vi "Main UI.vi"() -> ()   [LabVIEW 2013]
uses:
  <vilib>/Utility/miscctls.llb/LVRowAndColumnTypeDef.ctl
  <vilib>/Utility/miscctls.llb/LVRowAndColumnUnsignedTypeDef.ctl
  Sub vi/Global constant.vi
  <vilib>/regexp/Match Regular Expression.xnode
panel:
  out "Operator":string="A1644"
  out "W/O Qty":string="20000"
  out "Work Order":string="1644"
  out "Date Code (YYWW)":string="4416" caption="D/C (YYWW)"
  out "Lot Number (6 digits)":string="123456" caption="L/N (6 digits)"
  out "Part Number_Die Ver_Field":string="206CAH" caption="P/N_Die Ver_Field"
  out "FPY":cluster{"fail":u32, "pass":u32, "FPY":dbl}={"fail"=12345, "pass"=1234567, "FPY"=0.0} caption="FPY (Pass/Fail/Rate %)"
  out "Test Time":string
  in  "Cancel Button":bool
  out "SN":string
  out "Model":string
  out "Result":string
  in  "OK Button":bool
  in  "Multicolumn Listbox":i32(listbox)
  out "Horizontal Graduated Bar":u8(slide) max=28 scale=-1.0..7.0
  in  "Boolean 2":bool
  out "reslut":bool
  out "Boolean":bool
  out "?":string[](array[string])
  out "ItemTag":string
  # "Melexis Auto-Programming Machine\nFor MLX91206"
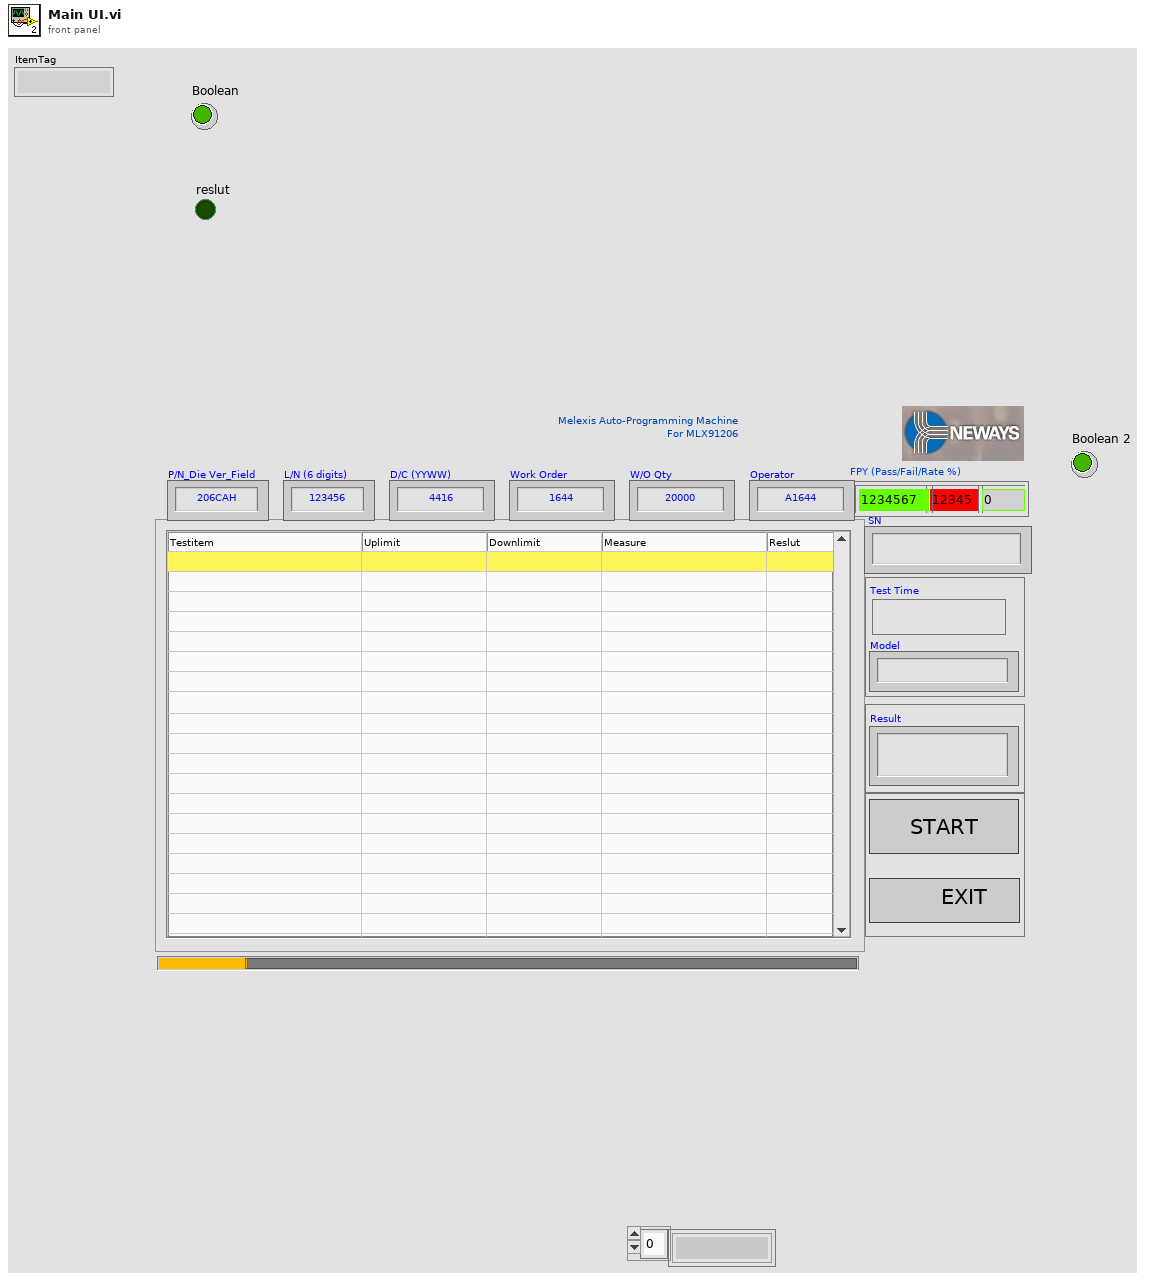
[diagram p1: front panel]
types:
  T1 = enum8{"Enabled", "Disabled", "Disabled and Grayed Out"}
  T2 = enum16{"open", "replace", "create", "open or create", "replace or create", "replace or create with confirmation"}
  T3 = typedef "LVRowAndColumnUnsignedTypeDef.ctl" = cluster{"Row":u32, "Column":u32}
  T4 = typedef "LVRowAndColumnTypeDef.ctl" = cluster{"Row":i32, "Column":i32}
  T5 = cluster{"step name 1":string, "updata 2":string, "limitdata 3":string, "load vi name 4":string, "parameter 5":string}
  T6 = cluster{"concatenated string":string, "Result":bool}
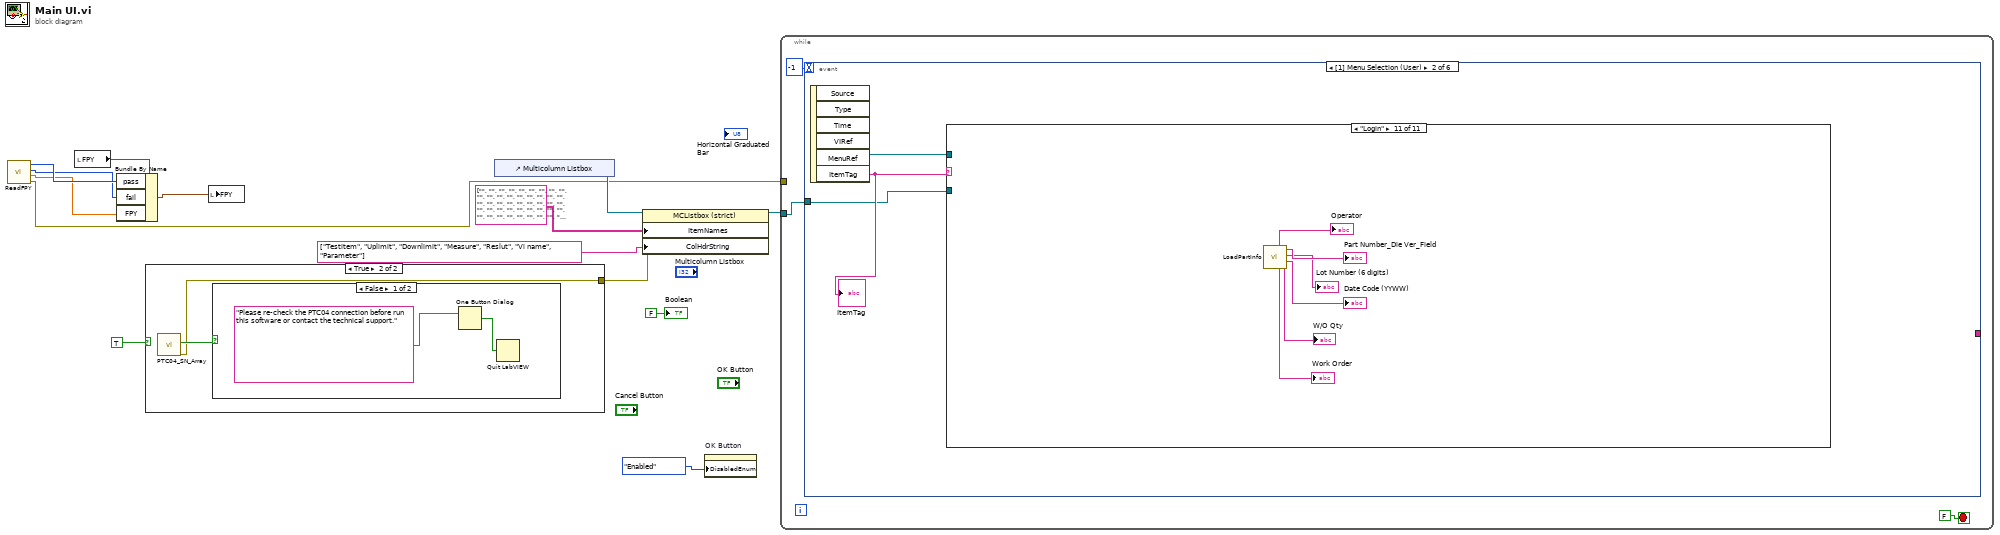
[diagram p0: block diagram]
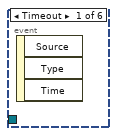
[diagram p4: hidden frame]
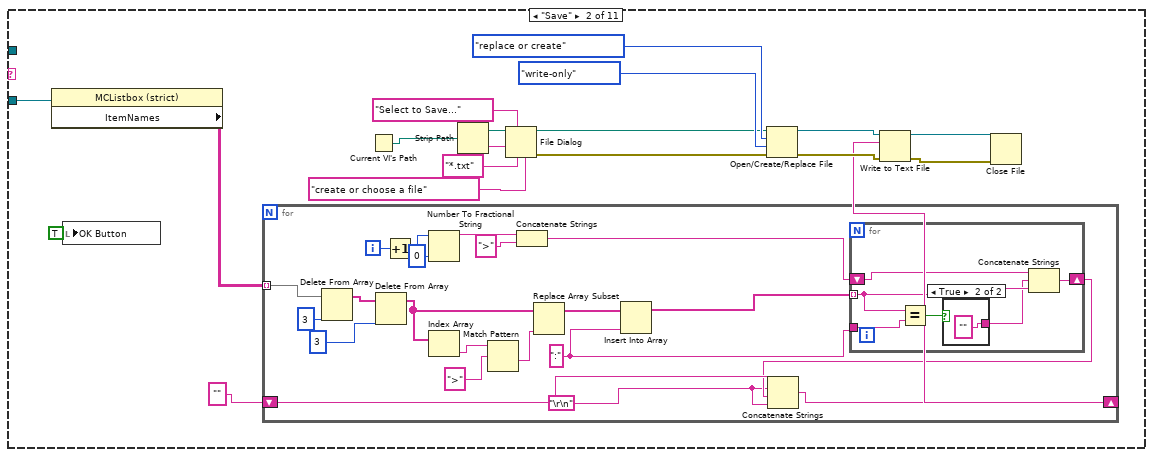
[diagram p6: hidden frame]
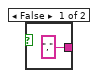
[diagram p7: hidden frame]
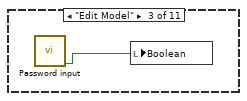
[diagram p8: hidden frame]
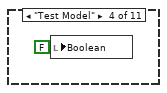
[diagram p9: hidden frame]
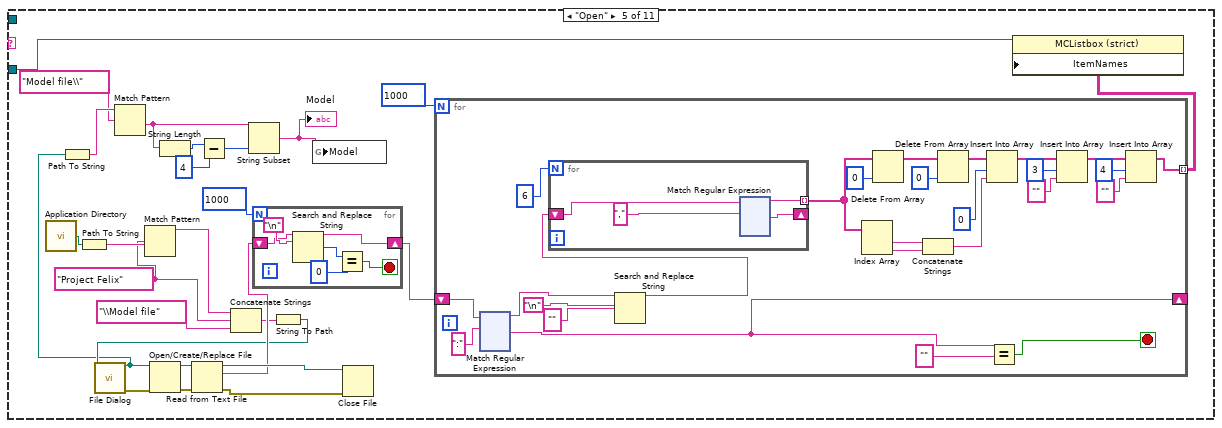
[diagram p10: hidden frame]
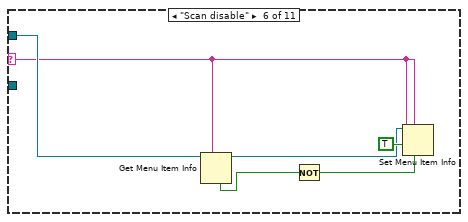
[diagram p11: hidden frame]
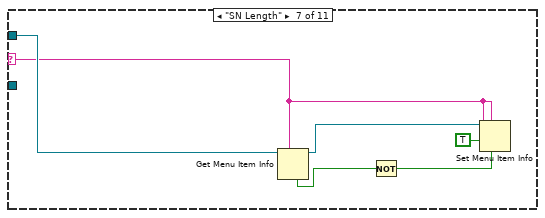
[diagram p12: hidden frame]
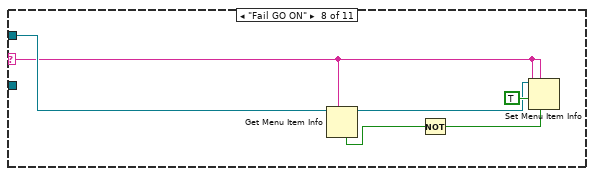
[diagram p13: hidden frame]
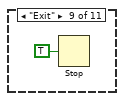
[diagram p14: hidden frame]
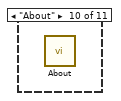
[diagram p15: hidden frame]
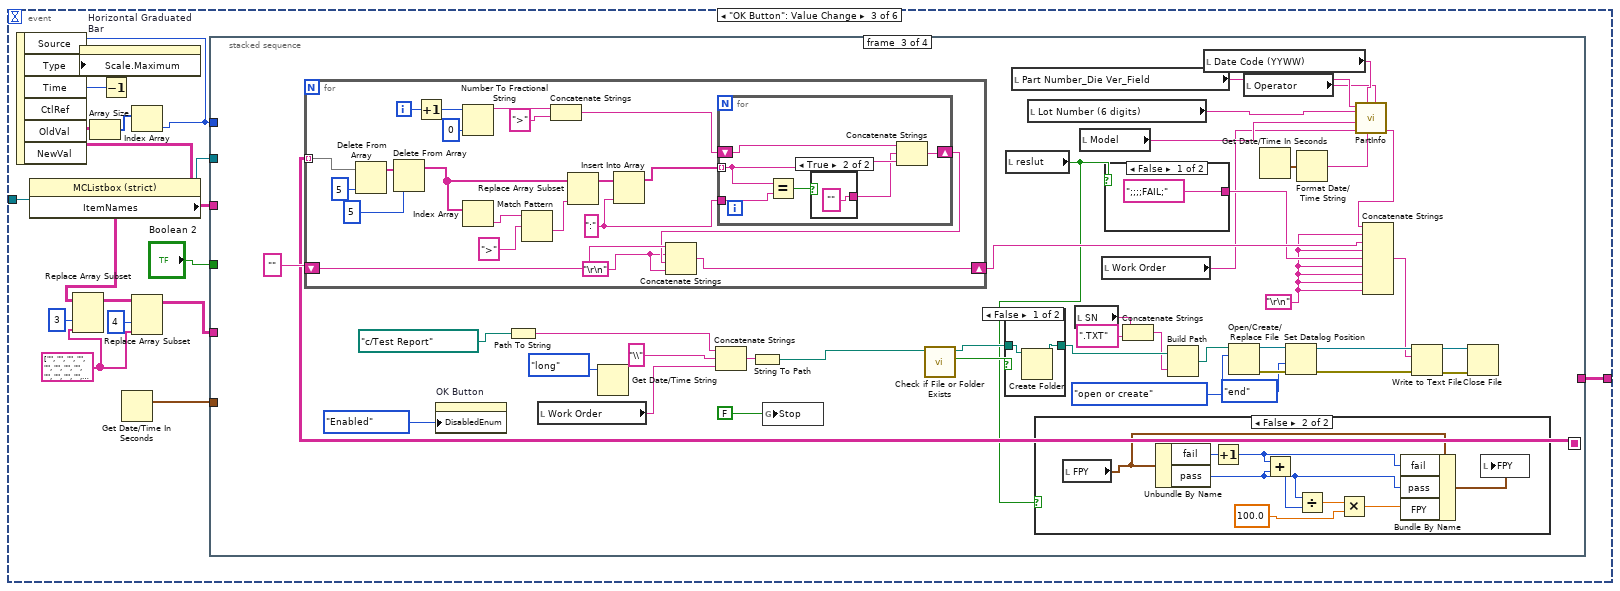
[diagram p16: hidden frame]
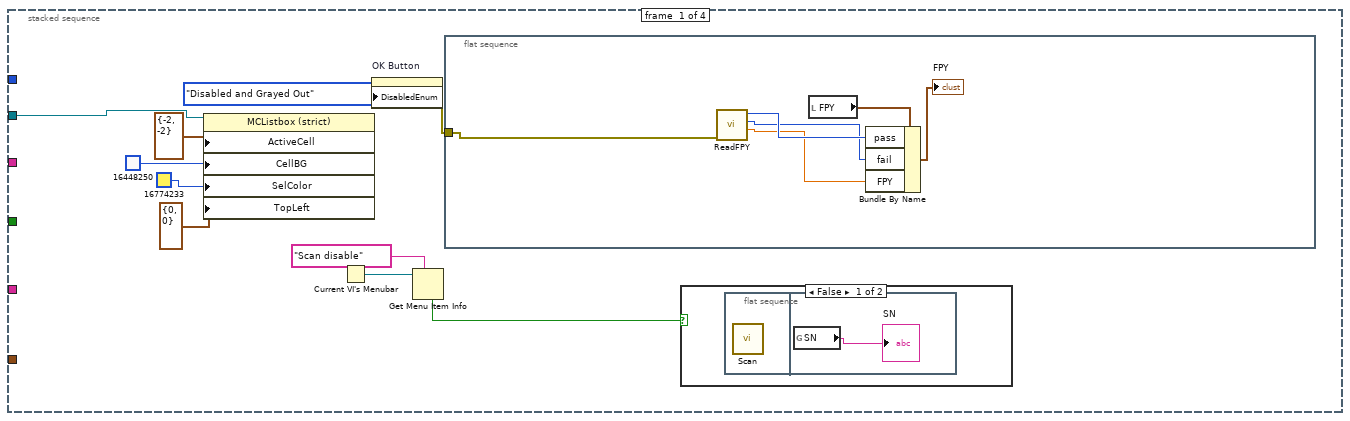
[diagram p17: hidden frame]
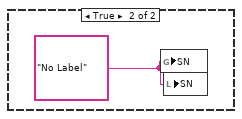
[diagram p18: hidden frame]
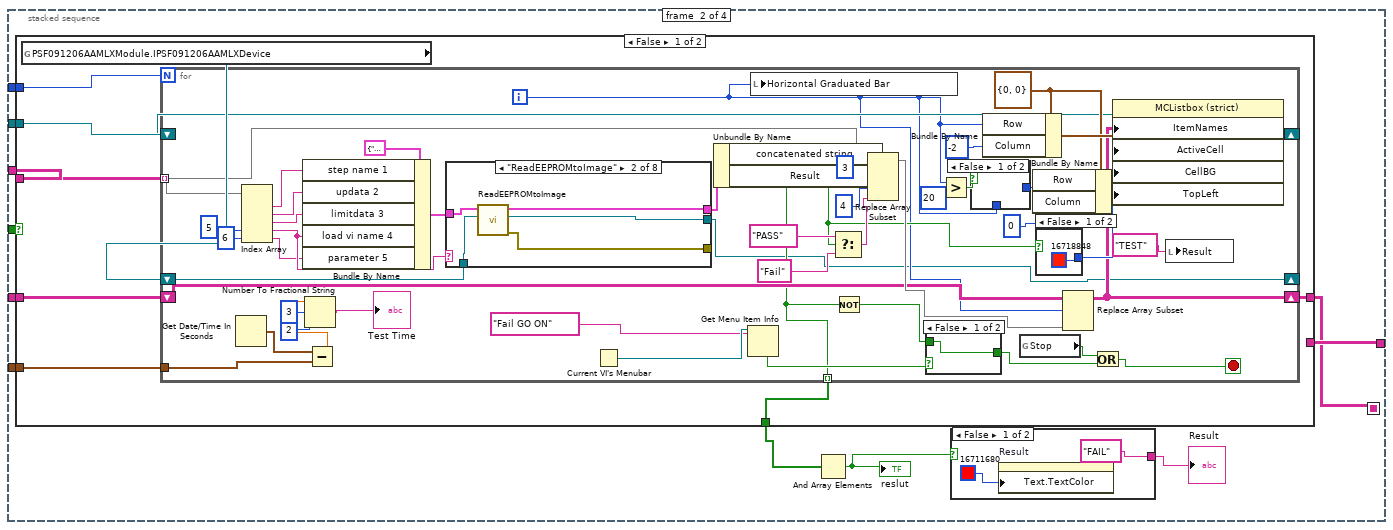
[diagram p19: hidden frame]
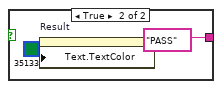
[diagram p20: hidden frame]
diagram:
  n1 = call "ReadFPY.vi"() -> ("error out"=w1:errorcluster, "FPY%"=w3:dbl, "fail"=w4:i32, "pass"=w5:i32)  [unwired: 7 in, 1 out]
  n2 = local read "FPY"() -> (w6:cluster{"fail":u32, "pass":u32, "FPY":dbl})
  n3 = Bundle By Name(cluster=w6, "pass"=w5, "fail"=w4, "FPY"=w3) -> (w2:cluster{"fail":u32, "pass":u32, "FPY":dbl})
  n4 = case shown="True" TRUE {
    tunnel: [_ w15] -> w7
    frame False {
    }
    frame True {
      n5 = call "PTC04_SN_Array.vi"() -> ("error out"=w15:errorcluster, "Register?"=w16:bool)  [unwired: 9 in, 1 out]
      n6 = case shown="False" w16 {
        frame False {
          n7 = One Button Dialog(message="Please re-check the PTC04 connection before run this software or contact the technical support.") -> (true=w17:bool)  [unwired: 1 in]
          n8 = Quit LabVIEW(quit? (T)=w17) -> ()
        }
        frame True {
        }
      }
    }
  }
  n9 = local write "FPY"(w2) -> ()
  n10 = control-ref of="Multicolumn Listbox"() -> (w14:refnum<vi>)
  n11 = property class="MCListbox (strict)"(reference=w14, error in=w7, "ItemNames"=string[][] [["", "", "", "", "", "", "", ""], ["", "", "", "", "", "", "", ""], ["", "", "", "", "", "", "", ""], ["", "", "", "", "", "", "", ""], ["", "", "", "", "", "", "", ""], ["", "", "", "", "", "", "", ""], ["", "", "", "", "", "", "", ""], ["", "", "", "", "", "", "", ""], ["", "", "", "", "", "", "", ""], ["", "", "", "", "", "", "", ""], ["", "", "", "", "", "", "", ""], ["", "", "", "", "", "", "", ""], ["", "", "", "", "", "", "", ""], ["", "", "", "", "", "", "", ""], ["", "", "", "", "", "", "", ""], ["", "", "", "", "", "", "", ""], ["", "", "", "", "", "", "", ""], ["", "", "", "", "", "", "", ""], ["", "", "", "", "", "", "", ""], ["", "", "", "", "", "", "", ""], ["", "", "", "", "", "", "", ""], ["", "", "", "", "", "", "", " "], ["", "", "", "", "", "", "", ""], ["", "", "", "", "", "", "", ""], ["", "", "", "", "", "", "", ""], ["", "", "", "", "", "", "", ""], ["", "", "", "", "", "", "", ""], ["", "", "", "", "", "", "", ""], ["", "", "", "", "", "", "", ""], ["", "", "", "", "", "", "", ""], ["", "", "", "", "", "", "", ""], ["", "", "", "", "", "", "", ""], ["", "", "", "", "", "", "", ""], ["", "", "", "", "", "", "", ""], ["", "", "", "", "", "", "", ""], ["", "", "", "", "", "", "", ""], ["", "", "", "", "", "", "", ""], ["", "", "", "", "", "", "", ""], ["", "", "", "", "", "", "", ""], ["", "", "", "", "", "", "", ""], ["", "", "", "", "", "", "", ""], ["", "", "", "", "", "", "", ""]] ("Item Names"), "ColHdrString"=string[] ["Testitem", "Uplimit", "Downlimit", "Measure", "Reslut", "Vi name", "Parameter"] ("Row Header Strings[]")) -> (reference out=w11:refnum<vi>)  [unwired: 1 out]
  n12 = property on="OK Button" class="Bool (strict)"("DisabledEnum"=T1."Enabled" ("Disabled")) -> ()  [unwired: 2 in, 2 out]
  n13 = while {
    tunnel: w11 -> [w21]
    tunnel: w1 -> [_]
    stop <- FALSE stop-if-true
    n14 = event shown="[1] Menu Selection (User)" {
      selector: _ -> [_ _ _ _ _ _]
      dyn-events: _ -> [_ _ _ _ _ _]
      timeout: -1 -> [_ _ _ _ _ _]
      tunnel: w21 -> [_ w23 w403 _ w712 w735]
      tunnel: [_ _ w390 _ _ _] -> _
      event Timeout {
        n15 = event-data() -> ()  [unwired: 1 in, 3 out]
      }
      event Menu Selection (User) {
        n16 = event-data() -> ("MenuRef"=w22:refnum<k9>, "ItemTag"=w24:string)  [unwired: 1 in, 4 out]
        "ItemTag" <- w24
        n17 = case shown="\"Login\"" w24 {
          selector: w24 -> [_ _ _ _ _ w365 w371 w380 _ _ _]
          tunnel: w23 -> [_ w43 _ _ w96 _ _ _ _ _ _]
          tunnel: w22 -> [_ _ _ _ _ w366 w372 w381 _ _ _]
          frame "False", Default {
          }
          frame "Save" {
            n18 = property class="MCListbox (strict)"(reference=w43) -> ("ItemNames"=w32:string[][])  [unwired: 1 in, 2 out]
            n19 = local write "OK Button"(TRUE ("OK Button")) -> ()
            n20 = for {
              tunnel: w32 -> [w54] mode=indexing
              shift-right: [w58] -> w29
              shift-left: "" -> [w57]
              i -> [w64]
              w44 = ":" ("new element/subarray")
              w55 = "\r\n"
              n21 = Delete From Array(array=w54, index=3) -> (array with subset deleted=w51:string[])  [unwired: 1 in, 1 out]
              n22 = Delete From Array(array=w51, index=3) -> (array with subset deleted=w49:string[])  [unwired: 1 in, 1 out]
              n23 = Increment(x=w64) -> (x+1=w63:i32)
              n24 = Number To Fractional String(number=w63, precision (6)=i16 0) -> (F-format string=w62:string)  [unwired: 2 in]
              n25 = Index Array(array=w49) -> (element=w50:string)  [unwired: 1 in]
              n26 = Match Pattern(string=w50, regular expression=">") -> (after substring=w48:string)  [unwired: 1 in, 3 out]
              n27 = Concatenate Strings(w62, ">") -> (w60:string)
              n28 = Replace Array Subset(array=w49, new element=w48) -> (w46:string[])  [unwired: 1 in]
              n29 = Insert Into Array(array=w46, new element=w44) -> (w45:string[])  [unwired: 1 in]
              n30 = for {
                shift-right: [w69] -> w56
                shift-left: w60 -> [w70]
                tunnel: w45 -> [w67] mode=indexing
                tunnel: w44 -> [w68]
                n31 = Equal?(x=w67, y=w68) -> (x = y?=w66:bool)
                n32 = case shown="True" w66 {
                  tunnel: ["," ("string") ""] -> w65
                  frame False {
                  }
                  frame True {
                  }
                }
                n33 = Concatenate Strings(w70, w65, w67) -> (w69:string)
              }
              n34 = Concatenate Strings(w57, w55, w56, w55) -> (w58:string)
            }
            n35 = Current VI's Path() -> (path=w26:path)
            n36 = Strip Path(path=w26) -> (stripped path=w34:path, name=w35:string)
            n37 = File Dialog(4:"create or choose a file" ("pattern label"), 6:"*.txt" ("pattern (all files)"), 7:"Select to Save..." ("prompt"), 9:w35, 11:w34) -> (0:w37:errorcluster, 3:w36:path)  [unwired: 1 in, 3 out]
            n38 = Open/Create/Replace File(file path (use dialog)=w36, error in=w37, operation (0:open)=T2."replace or create", access (0:read/write)=enum16{"read/write", "read-only", "write-only"}."write-only") -> (refnum out=w30:refnum<file>, error out=w31:errorcluster)  [unwired: 3 out]
            n39 = Write to Text File(file (use dialog)=w30, text=w29, error in=w31) -> (refnum out=w27:refnum<file>, error out=w28:errorcluster)  [unwired: 1 in, 1 out]
            n40 = Close File(refnum=w27, error in=w28) -> ()  [unwired: 2 out]
          }
          frame "Edit Model" {
            n41 = call "Password input.vi"() -> ("Boolean"=w73:bool)  [unwired: 10 in, 1 out]
            n42 = local write "Boolean"(w73) -> ()
          }
          frame "Test Model" {
            n43 = local write "Boolean"(FALSE ("Boolean")) -> ()
          }
          frame "Open" {
            w79 = "Project Felix" ("search string")
            n44 = call <vilib>:"Application Directory.vi"() -> ("Application Directory"=w82:path)
            n45 = Path To String(path=w82) -> (string=w81:string)
            n46 = Match Pattern(string=w81, regular expression=w79) -> (before substring=w80:string)  [unwired: 1 in, 3 out]
            n47 = Concatenate Strings(w80, w79, "\\Model file" ("string")) -> (w77:string)
            n48 = String To Path(string=w77) -> (path=w76:path)
            n49 = call "File Dialog"("start path"=w76) -> ("selected path"=w75:path, "error out"=w98:errorcluster)  [unwired: 11 in, 2 out]
            n50 = Path To String(path=w75) -> (string=w92:string)
            n51 = Match Pattern(string=w92, regular expression="Model file\\") -> (after substring=w87:string)  [unwired: 1 in, 3 out]
            n52 = Open/Create/Replace File(file path (use dialog)=w75, error in=w98) -> (refnum out=w99:refnum<file>, error out=w100:errorcluster)  [unwired: 4 in, 1 out]
            n53 = String Length(string=w87) -> (length=w90:i32)
            n54 = Read from Text File(file (use dialog)=w99, error in=w100) -> (refnum out=w93:refnum<file>, text=w85:string, error out=w94:errorcluster)  [unwired: 2 in, 1 out]
            n55 = Subtract(x=w90, y=4) -> (x-y=w88:i32)
            n56 = String Subset(string=w87, length (rest)=w88) -> (substring=w83:string)  [unwired: 1 in]
            "Model" <- w83
            n57 = for {
              N: 1000 -> [_]
              shift-right: [w104] -> w84
              shift-left: w85 -> [w105]
              stop <- w101 stop-if-true
              n58 = Search and Replace String(input string=w105, search string="\n") -> (result string=w104:string, number of replacements=w103:i32)  [unwired: 6 in, 2 out]
              n59 = Equal?(x=w103, y=0) -> (x = y?=w101:bool)
            }
            n60 = global write "Global constant.vi" "Model"(w83) -> ()
            n61 = Close File(refnum=w93, error in=w94) -> ()  [unwired: 2 out]
            n62 = for {
              N: 1000 -> [_]
              shift-right: [w113] -> _
              shift-left: w84 -> [w132]
              tunnel: [w114] -> w95 mode=indexing
              stop <- w111 stop-if-true
              n63 = xnode ("Match Regular Expression")("input string"=w132, "regular expression"=":") -> ("before match"=w110:string, "after match"=w113:string)  [unwired: 4 in, 3 out]
              n64 = Search and Replace String(input string=w110, search string="\n" ("Line Feed Constant"), replace string="" ("replace string (\"\")")) -> (result string=w107:string)  [unwired: 5 in, 3 out]
              n65 = for {
                N: 6 -> [_]
                shift-right: [w134] -> _
                shift-left: w107 -> [w135]
                tunnel: [w133] -> w127 mode=indexing
                n66 = xnode "Match Regular Expression"("input string"=w135, "regular expression"=",") -> ("before match"=w133:string, "after match"=w134:string)  [unwired: 4 in, 3 out]
              }
              n67 = Index Array(array=w127) -> (element #1=w128:string, element #2=w129:string)  [unwired: 2 in]
              n68 = Delete From Array(array=w127, index=0) -> (array with subset deleted=w126:string[])  [unwired: 1 in, 1 out]
              n69 = Concatenate Strings(w128, w129) -> (w122:string)
              n70 = Delete From Array(array=w126, index=0) -> (array with subset deleted=w123:string[])  [unwired: 1 in, 1 out]
              n71 = Insert Into Array(array=w123, index=0, new element=w122) -> (w120:string[])
              n72 = Equal?(x=w113, y="") -> (x = y?=w111:bool)
              n73 = Insert Into Array(array=w120, index=3, new element="" ("new element/subarray")) -> (w117:string[])
              n74 = Insert Into Array(array=w117, index=4, new element="" ("new element/subarray")) -> (w114:string[])
            }
            n75 = property class="MCListbox (strict)"(reference=w96, "ItemNames"=w95) -> ()  [unwired: 1 in, 2 out]
          }
          frame "Scan disable" {
            n76 = Get Menu Item Info(7:w365, 11:w366) -> (3:w367:refnum<k9>, 4:w369:bool)  [unwired: 1 in, 5 out]
            n77 = Not(x=w369) -> (.not. x?=w368:bool)
            n78 = Set Menu Item Info(6:w368, 7:w365, 9:TRUE ("enabled"), 10:w365, 11:w367) -> ()  [unwired: 2 in, 2 out]
          }
          frame "SN Length" {
            n79 = Get Menu Item Info(7:w371, 11:w372) -> (3:w373:refnum<k9>, 4:w375:bool)  [unwired: 1 in, 5 out]
            n80 = Not(x=w375) -> (.not. x?=w374:bool)
            n81 = Set Menu Item Info(6:w374, 7:w371, 9:TRUE ("enabled"), 10:w371, 11:w373) -> ()  [unwired: 2 in, 2 out]
          }
          frame "Fail GO ON" {
            n82 = Get Menu Item Info(7:w380, 11:w381) -> (3:w377:refnum<k9>, 4:w379:bool)  [unwired: 1 in, 5 out]
            n83 = Not(x=w379) -> (.not. x?=w378:bool)
            n84 = Set Menu Item Info(6:w378, 7:w380, 9:TRUE ("enabled"), 10:w380, 11:w377) -> ()  [unwired: 2 in, 2 out]
          }
          frame "Exit" {
            n85 = Stop(stop? (T)=TRUE) -> ()
          }
          frame "About" {
            n86 = call "About.vi"() -> ()  [unwired: 12 in]
          }
          frame "Login" {
            n87 = call "LoadPartInfo.vi"() -> ("W/O Qty"=→"W/O Qty":string, "Date Code (YYWW) 2"=→"Date Code (YYWW)":string, "Lot Number (6 digits) 2"=→"Lot Number (6 digits)":string, "Part Number_Die Ver_Field 2"=→"Part Number_Die Ver_Field":string, "Work Order 2"=→"Work Order":string, "Operator 2"=→"Operator":string)  [unwired: 6 in]
          }
        }
      }
      event "OK Button": Value Change {
        w400 = string[] ["", "", "", "", "", "", "", "", "", "", "", "", "", "", "", "", "", "", "", "", "", "", "", "", "", "", "", "", "", "", "", "", "", "", "", "", "", "", "", "", "", "", "", "", "", "", "", "", "", "", "", "", "", "", "", "", "", "", "", "", "", "", "", "", "", "", "", "", "", "", "", "", "", "", "", "", "", "", "", "", "", "", "", "", "", "", "", "", "", "", "", "", "", "", "", "", "", "", "", "", ""] ("new element/subarray")
        n88 = event-data() -> ()  [unwired: 1 in, 6 out]
        n89 = property class="MCListbox (strict)"(reference=w403) -> (reference out=w402:refnum<vi>, "ItemNames"=w395:string[][])  [unwired: 1 in, 1 out]
        n90 = Replace Array Subset(array=w395, new element=w400, index (col)=3 ("disabled index (col)")) -> (w399:string[][])  [unwired: 1 in]
        n91 = Array Size(array=w395) -> (size(s)=w396:i32[])
        n92 = Get Date/Time In Seconds() -> (seconds since 1Jan1904=w391:timestamp)
        n93 = Index Array(array=w396) -> (element=w392:i32)  [unwired: 1 in]
        n94 = Decrement(x=w392) -> (x-1=w393:i32)
        n95 = property on="Horizontal Graduated Bar" class="Slide (strict)"("Scale.Maximum"=w393) -> ()  [unwired: 2 in, 2 out]
        n96 = Replace Array Subset(array=w399, new element=w400, index (col)=4 ("disabled index (col)")) -> (w397:string[][])  [unwired: 1 in]
        n97 = stacked-sequence {
          seq-local: [_ w425 _ _] -> [_ _ w626 _]
          tunnel: w402 -> [w409 w429 _ _]
          tunnel: w392 -> [_ w432 _ _]
          tunnel: w397 -> [_ w431 _ _]
          tunnel: w395 -> [_ w430 _ _]
          tunnel: "Boolean 2" -> [_ w428 _ _]
          tunnel: w391 -> [_ w427 _ _]
          tunnel: [_ w426 _ _] -> w390
          frame #0 {
            n98 = property class="MCListbox (strict)"(reference=w409, "ActiveCell"=T4 {"Row"=-2, "Column"=-2} ("Active Cell:Active Cell"), "CellBG"=u32 16448250, "SelColor"=u32 16774233, "TopLeft"=T3 {"Row"=0, "Column"=0} ("Top Left Visible Cell")) -> ()  [unwired: 1 in, 2 out]
            n99 = Current VI's Menubar() -> (w412:refnum<k9>)
            n100 = property on="OK Button" class="Bool (strict)"("DisabledEnum"=T1."Disabled and Grayed Out" ("Disabled")) -> (error out=w404:errorcluster)  [unwired: 2 in, 1 out]
            n101 = Get Menu Item Info(7:"Scan disable" ("item tag"), 11:w412) -> (4:w410:bool)  [unwired: 1 in, 6 out]
            n102 = flat-sequence {
              tunnel: w404 -> [w417]
              frame #0 {
                n103 = call "ReadFPY.vi"("error in (no error)"=w417) -> ("FPY%"=w414:dbl, "fail"=w415:i32, "pass"=w416:i32)  [unwired: 6 in, 2 out]
                n104 = local read "FPY"() -> (w419:cluster{"fail":u32, "pass":u32, "FPY":dbl})
                n105 = Bundle By Name(cluster=w419, "pass"=w416, "fail"=w415, "FPY"=w414) -> (→"FPY":cluster{"fail":u32, "pass":u32, "FPY":dbl})
              }
            }
            n106 = case shown="False" w410 {
              frame False {
                n107 = flat-sequence {
                  frame #0 {
                    n108 = call "Scan.vi"() -> ()  [unwired: 12 in]
                  }
                  frame #1 {
                    n109 = global read "Global constant.vi" "SN"() -> (→"SN":string)
                  }
                }
              }
              frame True {
                w421 = "No Label"
                n110 = global write "Global constant.vi" "SN"(w421) -> ()
                n111 = local write "SN"(w421) -> ()
              }
            }
          }
          frame #1 {
            n112 = case shown="False" w428 {
              tunnel: w432 -> [w441 w545]
              tunnel: w431 -> [w444 w544]
              tunnel: w430 -> [w443 w543]
              tunnel: w429 -> [w442 w542]
              tunnel: [w440 w541] -> w422
              tunnel: w427 -> [w439 w540]
              tunnel: [_ w539] -> w426
              tunnel: [w438 _] -> w425
              frame False {
                n113 = global read "Global constant.vi" "PSF091206AAMLXModule.IPSF091206AAMLXDevice"() -> (w437:refnum<k7>)
                n114 = for {
                  N: w441 -> [_]
                  tunnel: w443 -> [w468] mode=indexing
                  shift-right: [w466] -> w438
                  shift-left: w444 -> [w467]
                  shift-right: [w465] -> _
                  shift-left: w442 -> [w469]
                  tunnel: [w462] -> w440 mode=indexing
                  tunnel: w439 -> [w459]
                  shift-right: [w446] -> _
                  shift-left: w437 -> [w445]
                  i -> [w461]
                  stop <- w449 stop-if-true
                  w476 = T4 {"Row"=0, "Column"=0} ("Active Cell:Active Cell")
                  n115 = Get Date/Time In Seconds() -> (seconds since 1Jan1904=w458:timestamp)
                  n116 = Index Array(array=w468, index #4=5 ("index"), index #5=6 ("index")) -> (element #1=w492:string, element #2=w491:string, element #3=w490:string, element #4=w453:string, element #5=w452:string)  [unwired: 3 in]
                  n117 = Bundle By Name(cluster=T5 {"step name 1"="", "updata 2"="", "limitdata 3"="", "load vi name 4"="", "parameter 5"=""} ("IN"), "step name 1"=w492, "updata 2"=w491, "limitdata 3"=w490, "load vi name 4"=w453, "parameter 5"=w452) -> (w489:T5)
                  n118 = Subtract(x=w458, y=w459) -> (x-y=w457:dbl)
                  n119 = Number To Fractional String(number=w457, width (-)=i16 3, precision (6)=i16 2) -> (F-format string=→"Test Time":string)  [unwired: 1 in]
                  n120 = case shown="\"ReadEEPROMtoImage\"" w453 {
                    tunnel: w489 -> [w504 w509 w513 w516 w521 w528 w533 w538]
                    tunnel: [w503 w508 w512 w518 w523 w526 w531 w536] -> _
                    tunnel: [w502 w507 w511 w517 w522 w527 w532 w537] -> w470
                    tunnel: [w501 w506 w510 w514 w520 w525 w530 w535] -> w446
                    tunnel: w445 -> [w501 w505 w510 w515 w519 w524 w529 w534]
                    frame "Init_Programmer" {
                      n121 = call "PTC04_SN_Array.vi"("IN"=w504) -> ("error out"=w503:errorcluster, "Cluster"=w502:T6)  [unwired: 8 in, 1 out]
                    }
                    frame "ReadEEPROMtoImage" {
                      n122 = call "ReadEEPROMtoImage.vi"("Automation Refnum"=w505, "IN"=w509) -> ("error out"=w508:errorcluster, "reference out"=w506:refnum<k7>, "Cluster"=w507:T6)  [unwired: 7 in]
                    }
                    frame "Delay_ms", Default {
                      n123 = call "Delay_ms.vi"("IN"=w513) -> ("error out"=w512:errorcluster, "Cluster"=w511:T6)  [unwired: 9 in]
                    }
                    frame "CopyImagetoTemp" {
                      n124 = call "CopyImagetoTemp.vi"("reference"=w515, "IN"=w516) -> ("error out"=w518:errorcluster, "reference out"=w514:refnum<k7>, "Cluster"=w517:T6)  [unwired: 7 in]
                    }
                    frame "SetRoughGainandFineGain" {
                      n125 = call "SetRoughGainandFineGain.vi"("reference"=w519, "IN"=w521) -> ("error out"=w523:errorcluster, "reference out"=w520:refnum<k7>, "Cluster"=w522:T6)  [unwired: 7 in]
                    }
                    frame "ReadRoughGainandFineGain" {
                      n126 = call "ReadRoughGainandFineGain.vi"("reference"=w524, "IN"=w528) -> ("error out"=w526:errorcluster, "reference out"=w525:refnum<k7>, "Cluster"=w527:T6)  [unwired: 7 in]
                    }
                    frame "ProgramEEPROMwithTemp" {
                      n127 = call "ProgramEEPROMwithTemp.vi"("reference"=w529, "IN"=w533) -> ("error out"=w531:errorcluster, "reference out"=w530:refnum<k7>, "Cluster"=w532:T6)  [unwired: 7 in]
                    }
                    frame "ReadEEPROMtoVerify" {
                      n128 = call "ReadEEPROMtoVerify.vi"("reference"=w534, "IN"=w538) -> ("error out"=w536:errorcluster, "reference out"=w535:refnum<k7>, "Cluster"=w537:T6)  [unwired: 7 in]
                    }
                  }
                  n129 = Current VI's Menubar() -> (w481:refnum<k9>)
                  n130 = Unbundle By Name(w470) -> ("concatenated string"=w487:string, "Result"=w462:bool)
                  n131 = Get Menu Item Info(7:"Fail GO ON" ("item tag"), 11:w481) -> (4:w464:bool)  [unwired: 1 in, 6 out]
                  n132 = local write "Horizontal Graduated Bar"(w461) -> ()
                  n133 = Select(t="PASS", s=w462, f="Fail") -> (s? t:f=w483:string)
                  n134 = Not(x=w462) -> (.not. x?=w463:bool)
                  n135 = Replace Array Subset(array=w468, new element #1=w487, index #1=3 ("index"), new element #2=w483, index #2=4 ("index")) -> (w482:string[])
                  n136 = case shown="False" w464 {
                    tunnel: [w494 FALSE] -> w448
                    tunnel: w463 -> [w494 _]
                    frame False {
                    }
                    frame True {
                    }
                  }
                  n137 = Greater?(x=w461, y=20) -> (0:w472:bool)
                  n138 = case shown="False" w472 {
                    tunnel: w461 -> [_ w498]
                    tunnel: [_ w496] -> w471
                    frame False {
                    }
                    frame True {
                      n139 = Subtract(x=w498, y=18) -> (x-y=w496:i32)
                    }
                  }
                  n140 = Bundle By Name(cluster=w476, "Row"=w461, "Column"=-2) -> (w477:T4)
                  n141 = global read "Global constant.vi" "Stop"() -> (w447:bool)
                  n142 = Bundle By Name(cluster=w476, "Row"=w471, "Column"=0) -> (w475:T4)
                  n143 = case shown="False" w462 {
                    tunnel: [u32 16718848 u32 65295] -> w479
                    frame False {
                    }
                    frame True {
                    }
                  }
                  n144 = Replace Array Subset(array=w467, new element=w482, index (row)=w461) -> (w466:string[][])  [unwired: 1 in]
                  n145 = Or(x=w447, y=w448) -> (x .or. y?=w449:bool)
                  n146 = property class="MCListbox (strict)"(reference=w469, "ItemNames"=w466, "ActiveCell"=w477, "CellBG"=w479, "TopLeft"=w475) -> (reference out=w465:refnum<vi>)  [unwired: 1 in, 1 out]
                  n147 = local write "Result"("TEST") -> ()
                }
              }
              frame True {
                n148 = for {
                  N: w545 -> [_]
                  tunnel: w543 -> [w593] mode=indexing
                  shift-right: [w590] -> w539
                  shift-left: w544 -> [w591]
                  tunnel: [w555] -> w541 mode=indexing
                  shift-right: [w579] -> _
                  shift-left: w542 -> [w578]
                  tunnel: w540 -> [w566]
                  i -> [w568]
                  stop <- w585 stop-if-true
                  w574 = T4 {"Row"=0, "Column"=0} ("Active Cell:Active Cell")
                  w581 = "Project Felix" ("regular expression")
                  n149 = call <vilib>:"Application Directory.vi"() -> ("Application Directory"=w584:path)
                  n150 = Path To String(path=w584) -> (string=w583:string)
                  n151 = Index Array(array=w593, index #1=5 ("index"), index #2=0 ("index"), index #3=1 ("index"), index #4=2 ("index"), index #5=6 ("index")) -> (element #1=w547:string, element #2=w551:string, element #3=w550:string, element #4=w549:string, element #5=w548:string)
                  n152 = Match Pattern(string=w583, regular expression=w581) -> (before substring=w582:string)  [unwired: 1 in, 3 out]
                  n153 = Get Date/Time In Seconds() -> (seconds since 1Jan1904=w565:timestamp)
                  n154 = Concatenate Strings(w582, w581) -> (w580:string)
                  n155 = Concatenate Strings(w580, "\\Test step\\" ("string"), w547, ".vi" ("string")) -> (w596:string)
                  n156 = Subtract(x=w565, y=w566) -> (x-y=w562:dbl)
                  n157 = String To Path(string=w596) -> (path=w558:path)
                  n158 = Bundle By Name(cluster=T5 {"step name 1"="", "updata 2"="", "limitdata 3"="", "load vi name 4"="", "parameter 5"=""} ("IN"), "step name 1"=w551, "updata 2"=w550, "limitdata 3"=w549, "load vi name 4"=w547, "parameter 5"=w548) -> (w546:T5)
                  n159 = Number To Fractional String(number=w562, width (-)=i16 3, precision (6)=i16 2) -> (F-format string=w561:string)  [unwired: 1 in]
                  n160 = local write "Horizontal Graduated Bar"(w568) -> ()
                  n161 = local write "Test Time"(w561) -> ()
                  n162 = Open VI Reference(type specifier VI Refnum (for type only)=refnum<vi> refnum, vi path=w558) -> (vi reference=w557:refnum<vi>)  [unwired: 4 in, 1 out]
                  n163 = call-by-ref "?"(reference=w557, "IN"=w546) -> ("Cluster"=w556:T6)  [unwired: 10 in, 3 out]
                  n164 = Unbundle By Name(w556) -> ("concatenated string"=w554:string, "Result"=w555:bool)
                  n165 = Current VI's Menubar() -> (w589:refnum<k9>)
                  n166 = Not(x=w555) -> (.not. x?=w586:bool)
                  n167 = Get Menu Item Info(7:"Fail GO ON" ("item tag"), 11:w589) -> (4:w587:bool)  [unwired: 1 in, 6 out]
                  n168 = Select(t="PASS", s=w555, f="Fail") -> (s? t:f=w600:string)
                  n169 = Replace Array Subset(array=w593, new element #1=w554, index #1=3 ("index"), new element #2=w600, index #2=4 ("index")) -> (w599:string[])
                  n170 = case shown="False" w587 {
                    tunnel: [w610 FALSE] -> w585
                    tunnel: w586 -> [w610 _]
                    frame False {
                    }
                    frame True {
                    }
                  }
                  n171 = case shown="True" w555 {
                    tunnel: [u32 16718848 u32 65295] -> w577
                    frame False {
                    }
                    frame True {
                    }
                  }
                  n172 = Greater?(x=w568, y=20) -> (0:w570:bool)
                  n173 = case shown="False" w570 {
                    tunnel: w568 -> [_ w607]
                    tunnel: [_ w605] -> w569
                    frame False {
                    }
                    frame True {
                      n174 = Subtract(x=w607, y=18) -> (x-y=w605:i32)
                    }
                  }
                  n175 = Bundle By Name(cluster=w574, "Row"=w568, "Column"=-2) -> (w575:T4)
                  n176 = Bundle By Name(cluster=w574, "Row"=w569, "Column"=0) -> (w573:T4)
                  n177 = Replace Array Subset "Replace Array Subset"(array=w591, new element=w599, index (row)=w568) -> (w590:string[][])  [unwired: 1 in]
                  n178 = property class="MCListbox (strict)"(reference=w578, "ItemNames"=w590, "ActiveCell"=w575, "CellBG"=w577, "TopLeft"=w573) -> (reference out=w579:refnum<vi>)  [unwired: 1 in, 1 out]
                  n179 = local write "Result"("TEST") -> ()
                }
              }
            }
            n180 = And Array Elements(Boolean array=w422) -> (logical AND=w423:bool)
            "reslut" <- w423
            n181 = case shown="False" w423 {
              tunnel: ["FAIL" "PASS"] -> w424
              frame False {
                n182 = property on="Result" class="Str"("Text.TextColor"=u32 16711680) -> ()  [unwired: 2 in, 2 out]
              }
              frame True {
                n183 = property on="Result" class="Str"("Text.TextColor"=u32 35133) -> ()  [unwired: 2 in, 2 out]
              }
            }
            "Result" <- w424
          }
          frame #2 {
            w615 = "\r\n"
            n184 = for {
              tunnel: w626 -> [w677] mode=indexing
              shift-right: [w689] -> w633
              shift-left: "" -> [w688]
              i -> [w695]
              w678 = ":" ("new element/subarray")
              w686 = "\r\n"
              n185 = Delete From Array(array=w677, index=5) -> (array with subset deleted=w676:string[])  [unwired: 1 in, 1 out]
              n186 = Delete From Array(array=w676, index=5) -> (array with subset deleted=w675:string[])  [unwired: 1 in, 1 out]
              n187 = Increment(x=w695) -> (x+1=w694:i32)
              n188 = Number To Fractional String(number=w694, precision (6)=i16 0) -> (F-format string=w693:string)  [unwired: 2 in]
              n189 = Index Array(array=w675) -> (element=w683:string)  [unwired: 1 in]
              n190 = Match Pattern(string=w683, regular expression=">") -> (after substring=w682:string)  [unwired: 1 in, 3 out]
              n191 = Concatenate Strings(w693, ">") -> (w691:string)
              n192 = Replace Array Subset(array=w675, new element=w682) -> (w680:string[])  [unwired: 1 in]
              n193 = Insert Into Array(array=w680, new element=w678) -> (w679:string[])  [unwired: 1 in]
              n194 = for {
                shift-right: [w700] -> w687
                shift-left: w691 -> [w701]
                tunnel: w679 -> [w698] mode=indexing
                tunnel: w678 -> [w699]
                n195 = Equal?(x=w698, y=w699) -> (x = y?=w697:bool)
                n196 = case shown="True" w697 {
                  tunnel: ["," ("string") ""] -> w696
                  frame False {
                  }
                  frame True {
                  }
                }
                n197 = Concatenate Strings(w701, w696, w698) -> (w700:string)
              }
              n198 = Concatenate Strings(w688, w686, w687, w686) -> (w689:string)
            }
            n199 = property on="OK Button" class="Bool (strict)"("DisabledEnum"=T1."Enabled" ("Disabled")) -> ()  [unwired: 2 in, 2 out]
            n200 = Path To String(path=path "c:/Test Report" ("base path")) -> (string=w625:string)
            n201 = local read "Work Order"() -> (w612:string)
            n202 = Get Date/Time String(date format (0)=enum16{"short", "long", "abbreviated"}."long") -> ()  [unwired: 2 in, 2 out]
            n203 = Concatenate Strings(w625, "\\", w612) -> (w647:string)
            n204 = String To Path(string=w647) -> (path=w646:path)
            n205 = global write "Global constant.vi" "Stop"(FALSE) -> ()
            n206 = call <vilib>:"Check if File or Folder Exists.vi"("path"=w646) -> ("file or folder exists?"=w645:bool, "dup path"=w644:path)  [unwired: 8 in, 1 out]
            n207 = case shown="False" w645 {
              tunnel: w644 -> [w673 w674]
              tunnel: [w672 w674] -> w643
              frame False {
                n208 = Create Folder(path (use dialog)=w673) -> (created path=w672:path)  [unwired: 2 in, 2 out]
              }
              frame True {
              }
            }
            n209 = local read "reslut"() -> (w622:bool)
            n210 = local read "Part Number_Die Ver_Field"() -> (w619:string)
            n211 = local read "Lot Number (6 digits)"() -> (w618:string)
            n212 = case shown="False" w622 {
              frame True {
                n213 = local read "FPY"() -> (w659:cluster{"fail":u32, "pass":u32, "FPY":dbl})
                n214 = Unbundle By Name(w659) -> ("fail"=w657:u32, "pass"=w660:u32)
                n215 = Increment(x=w660) -> (x+1=w656:u32)
                n216 = Add(x=w657, y=w656) -> (x+y=w655:u32)
                n217 = Divide(x=w656, y=w655) -> (x/y=w654:dbl)
                n218 = Multiply(x=w654, y=100.0) -> (x*y=w653:dbl)
                n219 = Bundle By Name(cluster=w659, "fail"=w657, "pass"=w656, "FPY"=w653) -> (w658:cluster{"fail":u32, "pass":u32, "FPY":dbl})
                n220 = local write "FPY"(w658) -> ()
              }
              frame False {
                n221 = local read "FPY"() -> (w669:cluster{"fail":u32, "pass":u32, "FPY":dbl})
                n222 = Unbundle By Name(w669) -> ("fail"=w667:u32, "pass"=w662:u32)
                n223 = Increment(x=w667) -> (x+1=w661:u32)
                n224 = Add(x=w661, y=w662) -> (x+y=w666:u32)
                n225 = Divide(x=w662, y=w666) -> (x/y=w665:dbl)
                n226 = Multiply(x=w665, y=100.0) -> (x*y=w664:dbl)
                n227 = Bundle By Name(cluster=w669, "fail"=w661, "pass"=w662, "FPY"=w664) -> (w668:cluster{"fail":u32, "pass":u32, "FPY":dbl})
                n228 = local write "FPY"(w668) -> ()
              }
            }
            n229 = local read "SN"() -> (w630:string)
            n230 = local read "Model"() -> (w620:string)
            n231 = local read "Work Order"() -> (w614:string)
            n232 = case shown="False" w622 {
              tunnel: [";;;;FAIL;" ";;;;PASS;"] -> w632
              frame False {
              }
              frame True {
              }
            }
            n233 = Concatenate Strings(w630, ".TXT" ("string")) -> (w628:string)
            n234 = Build Path(base path=w643, name or relative path=w628) -> (appended path=w642:path)
            n235 = local read "Date Code (YYWW)"() -> (w617:string)
            n236 = Open/Create/Replace File(file path (use dialog)=w642, operation (0:open)=T2."open or create") -> (refnum out=w639:refnum<file>, error out=w640:errorcluster)  [unwired: 4 in, 1 out]
            n237 = local read "Operator"() -> (w613:string)
            n238 = Get Date/Time In Seconds() -> (seconds since 1Jan1904=w627:timestamp)
            n239 = Set Datalog Position(4:w640, 5:enum16{"start", "end", "current"}."end" ("from (0:start)"), 7:w639) -> (0:w636:errorcluster, 3:w637:refnum<file>)  [unwired: 1 in]
            n240 = Format Date/Time String(seconds (now)=w627) -> (date/time string=w621:string)  [unwired: 2 in]
            n241 = call "PartInfo.vi"("OP"=w613, "Time"=w621, "Date Code"=w617, "W/O"=w614, "model"=w620, "Lot#"=w618, "P/N"=w619) -> ("output string"=w616:string)  [unwired: 4 in]
            n242 = Concatenate Strings(w616, w615, w633, w615, w632, w615, w615, w615, w615) -> (w631:string)
            n243 = Write to Text File(file (use dialog)=w637, text=w631, error in=w636) -> (refnum out=w634:refnum<file>, error out=w635:errorcluster)  [unwired: 1 in, 1 out]
            n244 = Close File(refnum=w634, error in=w635) -> ()  [unwired: 2 out]
          }
          frame #3 {
            n245 = local read "FPY"() -> (w706:cluster{"fail":u32, "pass":u32, "FPY":dbl})
            n246 = Unbundle By Name(w706) -> ("pass"=w705:u32, "fail"=w704:u32)
            n247 = call "WriteFPY.vi"("fail"=w704, "pass"=w705) -> ()  [unwired: 9 in, 1 out]
          }
        }
      }
      event "Cancel Button": Value Change {
        n248 = event-data() -> ()  [unwired: 1 in, 6 out]
        n249 = flat-sequence {
          frame #0 {
            # "CLOSE ALL"
            n250 = global write "Global constant.vi" "Stop"(TRUE) -> ()
          }
          frame #1 {
            n251 = Two Button Dialog(message="Close the Window?") -> (T button?=w708:bool)  [unwired: 2 in]
            n252 = case shown="True" w708 {
              frame False {
              }
              frame True {
                n253 = control-ref of="This VI"() -> (w710:refnum<vi>)
                n254 = invoke class="VI" method="FP.Close"(reference=w710) -> ()  [unwired: 2 in, 3 out]
              }
            }
          }
        }
      }
      event "Multicolumn Listbox": Double Click {
        n255 = event-data() -> ()  [unwired: 1 in, 9 out]
        n256 = local read "Boolean"() -> (w711:bool)
        n257 = case shown="True" w711 {
          tunnel: w712 -> [_ w733]
          frame False {
          }
          frame True {
            n258 = property class="MCListbox (strict)"(reference=w733) -> (reference out=w726:refnum<vi>, "ItemNames"=w723:string[][], "Value"=w724:i32)  [unwired: 1 in, 1 out]
            n259 = Index Array(array=w723, index (row)=w724) -> (element=w732:string[])  [unwired: 1 in]
            n260 = Index Array(array=w732) -> (element #1=w730:string, element #2=w729:string, element #3=w728:string, element #6=w727:string, element #7=w713:string)  [unwired: 7 in, 2 out]
            n261 = Bundle By Name(cluster=T5 {"step name 1"="", "updata 2"="", "limitdata 3"="", "load vi name 4"="", "parameter 5"=""} ("IN"), "step name 1"=w730, "updata 2"=w729, "limitdata 3"=w728, "load vi name 4"=w727, "parameter 5"=w713) -> (w721:T5)
            n262 = call "Parameter Setting.vi"("TEST INFO"=w721) -> ("IN 2"=w722:T5)  [unwired: 10 in]
            n263 = Cluster To Array(cluster=w722) -> (array=w720:string[])
            n264 = Insert Into Array(array=w720, index=3, new element="" ("new element/subarray")) -> (w718:string[])
            n265 = Insert Into Array(array=w718, index=4, new element="" ("new element/subarray")) -> (w714:string[])
            n266 = Replace Array Subset(array=w723, new element=w714, index (row)=w724) -> (w725:string[][])  [unwired: 1 in]
            n267 = property class="MCListbox (strict)"(reference=w726, "ItemNames"=w725) -> ()  [unwired: 1 in, 2 out]
          }
        }
      }
      event "Multicolumn Listbox": Shortcut Menu Selection (User) {
        n268 = event-data() -> ("ItemTag"=w736:string)  [unwired: 1 in, 7 out]
        n269 = local read "Boolean"() -> (w734:bool)
        n270 = case shown="True" w734 {
          tunnel: w736 -> [_ w738]
          tunnel: w735 -> [_ w737]
          frame False {
          }
          frame True {
            n271 = case shown="\"COM\"" w738 {
              tunnel: w737 -> [w744 w745 w751 w760 w764 w771]
              frame "A", Default {
                n272 = property class="MCListbox (strict)"(reference=w744) -> (reference out=w743:refnum<vi>, "Value"=w742:i32, "ItemNames"=w739:string[][])  [unwired: 1 in, 1 out]
                n273 = Insert Into Array(array=w739, index (row)=w742, new element=string[] ["A45", "A", "A4", "66AAA", "AA"] ("new element/subarray")) -> (w740:string[][])  [unwired: 1 in]
                n274 = property class="MCListbox (strict)"(reference=w743, "ItemNames"=w740) -> ()  [unwired: 1 in, 2 out]
              }
              frame "B" {
                n275 = property class="MCListbox (strict)"(reference=w745) -> (reference out=w750:refnum<vi>, "Value"=w749:i32, "ItemNames"=w746:string[][])  [unwired: 1 in, 1 out]
                n276 = Insert Into Array(array=w746, index (row)=w749, new element=string[] ["B45", "B", "B4", "BBBBB6AAA", "BBBBBBA"] ("new element/subarray")) -> (w747:string[][])  [unwired: 1 in]
                n277 = property class="MCListbox (strict)"(reference=w750, "ItemNames"=w747) -> ()  [unwired: 1 in, 2 out]
              }
              frame "COM" {
                n278 = property class="MCListbox (strict)"(reference=w751) -> (reference out=w756:refnum<vi>, "Value"=w755:i32, "ItemNames"=w752:string[][])  [unwired: 1 in, 1 out]
                n279 = Insert Into Array(array=w752, index (row)=w755, new element=string[] ["COM1", "H", "L", "", ""] ("new element/subarray")) -> (w753:string[][])  [unwired: 1 in]
                n280 = property class="MCListbox (strict)"(reference=w756, "ItemNames"=w753) -> ()  [unwired: 1 in, 2 out]
              }
              frame "Paste" {
                n281 = property class="MCListbox (strict)"(reference=w760) -> (reference out=w758:refnum<vi>, "Value"=w761:i32, "ItemNames"=w762:string[][])  [unwired: 1 in, 1 out]
                n282 = local read item#2() -> (w759:string[])
                n283 = Replace Array Subset(array=w762, new element=w759, index (row)=w761) -> (w757:string[][])  [unwired: 1 in]
                n284 = property class="MCListbox (strict)"(reference=w758, "ItemNames"=w757) -> ()  [unwired: 1 in, 2 out]
              }
              frame "Delete" {
                n285 = property class="MCListbox (strict)"(reference=w764) -> (reference out=w767:refnum<vi>, "Value"=w763:i32, "ItemNames"=w765:string[][])  [unwired: 1 in, 1 out]
                n286 = Delete From Array(array=w765, index (row)=w763) -> (array with subset deleted=w766:string[][])  [unwired: 2 in, 1 out]
                n287 = property class="MCListbox (strict)"(reference=w767, "ItemNames"=w766) -> ()  [unwired: 1 in, 2 out]
              }
              frame "Copy" {
                n288 = property class="MCListbox (strict)"(reference=w771) -> ("Value"=w769:i32, "ItemNames"=w770:string[][])  [unwired: 1 in, 2 out]
                n289 = Index Array(array=w770, index (row)=w769) -> (element=→"?":string[])  [unwired: 1 in]
              }
            }
          }
        }
      }
    }
  }
  "Boolean" <- FALSE ("Boolean")
